vi "Module.vi"() -> ()   [LabVIEW 2022 SP3, in "Demo.lvlib"]
uses:
  Demo.lvlib
  Shared/Controls/Global.ctl
  Shared/Shared.lvlib
panel:
  out "Application:All VIs In Memory":string[](array[string])
  out "Application:All Libraries in Application Instance":string[](array[string])
  out "Ticks":u32
  out "Instances":T1[](array[typedef])
  out "Self":T1
  in  "_Exit":bool
  in  "ID":i32
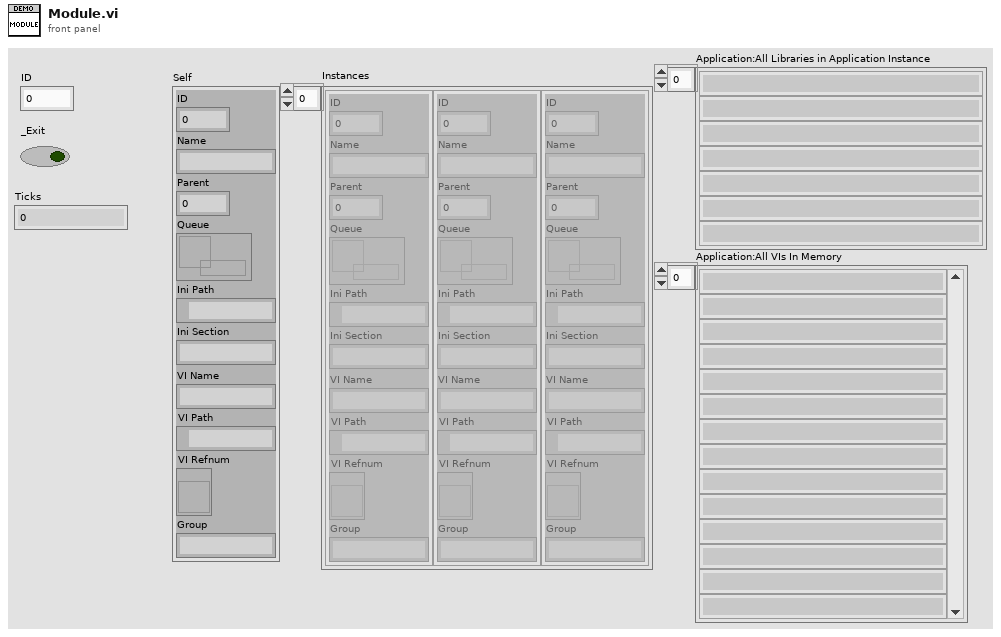
[diagram p1: front panel]
types:
  T1 = typedef "Shared.lvlib/Global.ctl" = cluster{"ID":i32, "Name":string, "Parent":i32, "Queue":refnum<queue>, "Ini Path":path, "Ini Section":string, "VI Name":string, "VI Path":path, "VI Refnum":refnum<vi>, "Group":string}
  T2 = typedef "Shared.lvlib/Instance.ctl" = cluster{"ID":i32, "Queue":refnum<queue>, "Global":refnum<k1>}
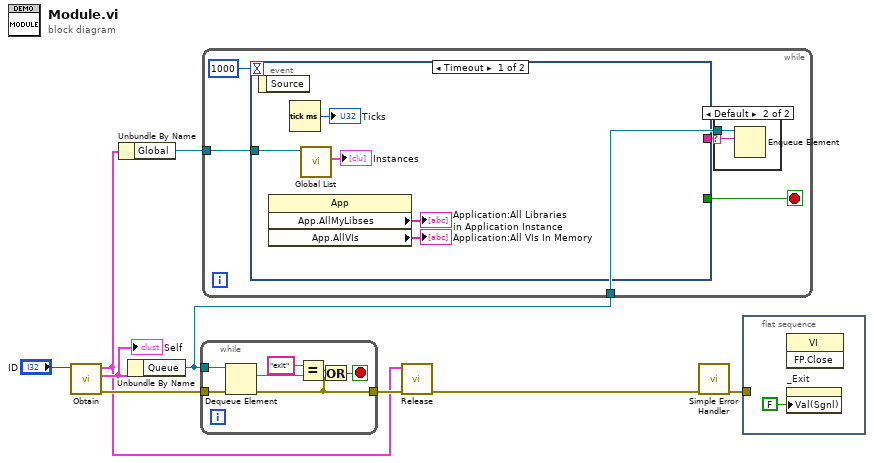
[diagram p0: block diagram]
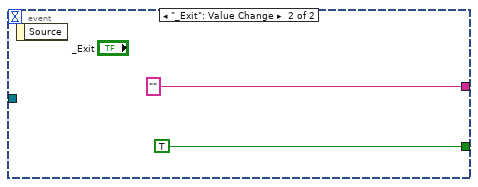
[diagram p3: hidden frame]
diagram:
  n1 = call "Obtain.vi"("ID in"="ID") -> ("error out"=w7:errorcluster, "Self"=w6:T1, "Instance"=w4:T2)  [unwired: 8 in]
  "Self" <- w6
  n2 = Unbundle By Name(w4) -> ("Global"=w3:refnum<k1>)
  n3 = Unbundle By Name(w6) -> ("Queue"=w5:refnum<queue>)
  n4 = while {
    tunnel: w5 -> [w16]
    tunnel: w7 -> [w15]
    tunnel: [w10] -> w8
    stop <- w11 stop-if-true
    n5 = Dequeue Element(queue=w16, error in (no error)=w15) -> (element=w14:string, error out=w10:errorcluster)  [unwired: 1 in, 2 out]
    n6 = Equal?(x="exit" ("y"), y=w14) -> (x = y?=w12:bool)
    n7 = Or(x=w12, y=w10) -> (x .or. y?=w11:bool)
  }
  n8 = while {
    tunnel: w5 -> [w21]
    tunnel: w3 -> [w17]
    stop <- w20 stop-if-true
    n9 = event shown="[0] Timeout" {
      selector: _ -> [_ _]
      dyn-events: _ -> [_ _]
      timeout: 1000 -> [_ _]
      tunnel: [_ TRUE] -> w20
      tunnel: [_ "" ("element")] -> w19
      tunnel: w17 -> [w28 _]
      event Timeout {
        n10 = event-data() -> ()  [unwired: 1 in, 1 out]
        n11 = property class="App"() -> ("App.AllMyLibses"=→"Application:All Libraries in Application Instance":string[], "App.AllVIs"=→"Application:All VIs In Memory":string[])  [unwired: 2 in, 2 out]
        n12 = Tick Count (ms)() -> (millisecond timer value=→"Ticks":u32)
        n13 = call "Global List.vi"("Global in"=w28) -> ("Instances"=→"Instances":T1[])  [unwired: 8 in, 2 out]
      }
      event "_Exit": Value Change {
        n14 = event-data() -> ()  [unwired: 1 in, 1 out]
      }
    }
    n15 = case shown="Default" w19 {
      selector: w19 -> [_ w22]
      tunnel: w21 -> [_ w23]
      frame "" {
      }
      frame Default {
        n16 = Enqueue Element(queue=w23, element=w22) -> ()  [unwired: 2 in, 3 out]
      }
    }
  }
  n17 = call "Release.vi"("error in (no error)"=w8, "Instance"=w4) -> ("error out"=w2:errorcluster)  [unwired: 8 in, 1 out]
  n18 = call <vilib>:"Simple Error Handler.vi"("error in (no error)"=w2) -> ("error out"=w1:errorcluster)  [unwired: 4 in, 4 out]
  n19 = flat-sequence {
    tunnel: w1 -> [_]
    frame #0 {
      n20 = invoke class="VI" method="FP.Close"() -> ()  [unwired: 3 in, 3 out]
      n21 = property on="_Exit" class="Bool (strict)"("Val(Sgnl)"=FALSE ("Value (Signaling)")) -> ()  [unwired: 2 in, 2 out]
    }
  }
